vi "initialise variables.vi"(11 "Data in":T1={"Parameters"={"FPGA Ref"=refnum, "data stream"={"data writer name"="error writer", "NS write buffer size"=16, "NS Buffer length"=0}, "FIFO Depth"=0, "Channel controls"={"FIFO channel count"=0, "active indices"=[], "active channels"=0, "channelScaling"=[], "scanivalveCount"=0, "channels"=[]}, "safetyChannels"={"oilP"=0, "airP"=0, "water"=0, "channelLimits"=[]}, "speedChannel"=0, "maxSpeedLimit"=0.0, "Torque"={"fixedOffset"=0.0, "filter"=FALSE, "fallingEdge"=FALSE, "swapEncoders"=FALSE}}, "Variables"={"Intermediary buffer"=[], "buffer position"=0, "write loop counter"=0, "NS write trigger"=0, "NS Connection status"=FALSE, "waiting for NS"=FALSE, "labAmbient"={"pressure"=0.0, "temperature"=0.0}, "scanivalvePorts"=[], "scanivalvePressures"=[], "data stream"="", "activeChannelLimitIndex"=[], "runningSpeedLimit"=0.0, "speedChannelIndex"=0, "Interlocks"={"gearboxOil"=FALSE, "bearingOil"=FALSE, "gearboxAir"=FALSE}, "interlockChannels"={"gearboxOil"=0, "bearingOil"=0, "air"=0}, "limitStates"=[]}}) -> (3 "Data out":T1={"Parameters"={"FPGA Ref"=refnum, "data stream"={"data writer name"="error writer", "NS write buffer size"=16, "NS Buffer length"=0}, "FIFO Depth"=0, "Channel controls"={"FIFO channel count"=0, "active indices"=[], "active channels"=0, "channelScaling"=[], "scanivalveCount"=0, "channels"=[]}, "safetyChannels"={"oilP"=0, "airP"=0, "water"=0, "channelLimits"=[]}, "speedChannel"=0, "maxSpeedLimit"=0.0, "Torque"={"fixedOffset"=0.0, "filter"=FALSE, "fallingEdge"=FALSE, "swapEncoders"=FALSE}}, "Variables"={"Intermediary buffer"=[], "buffer position"=0, "write loop counter"=0, "NS write trigger"=0, "NS Connection status"=FALSE, "waiting for NS"=FALSE, "labAmbient"={"pressure"=0.0, "temperature"=0.0}, "scanivalvePorts"=[], "scanivalvePressures"=[], "data stream"="", "activeChannelLimitIndex"=[], "runningSpeedLimit"=0.0, "speedChannelIndex"=0, "Interlocks"={"gearboxOil"=FALSE, "bearingOil"=FALSE, "gearboxAir"=FALSE}, "interlockChannels"={"gearboxOil"=0, "bearingOil"=0, "air"=0}, "limitStates"=[]}})   [LabVIEW 2018]
uses:
  Type Defs/Data processing loop data.ctl
  Type Defs/FPGA reference.ctl
  PC/type defs/channelControl.ctl
  Type Defs/channelScalingTypes.ctl
  Type Defs/scalingMethods.ctl
  ICL-LabVIEW_General/data channels/parent class/Data Channel.lvclass
  PC/type defs/channelLimitControl.ctl
  PC/type defs/limitActions.ctl
  Type Defs/channelConfigFilePath.ctl
  ICL-LabVIEW_General/data channels/data channels.lvlib
types:
  T1 = typedef "Data processing loop data.ctl" = cluster{"Parameters":cluster{"FPGA Ref":T2, "data stream":cluster{"data writer name":string, "NS write buffer size":i32, "NS Buffer length":u32}, "FIFO Depth":u32, "Channel controls":cluster{"FIFO channel count":i32, "active indices":i16[], "active channels":i32, "channelScaling":T3[], "scanivalveCount":i32, "channels":refnum<class "Data Channel.lvclass">[]}, "safetyChannels":cluster{"oilP":u16, "airP":u16, "water":u16, "channelLimits":T6[]}, "speedChannel":i32, "maxSpeedLimit":dbl, "Torque":cluster{"fixedOffset":dbl, "filter":bool, "fallingEdge":bool, "swapEncoders":bool}}, "Variables":cluster{"Intermediary buffer":dbl[][], "buffer position":u32, "write loop counter":u16, "NS write trigger":u32, "NS Connection status":bool, "waiting for NS":bool, "labAmbient":cluster{"pressure":dbl, "temperature":dbl}, "scanivalvePorts":u16[], "scanivalvePressures":dbl[], "data stream":refnum<k21>, "activeChannelLimitIndex":u16[], "runningSpeedLimit":dbl, "speedChannelIndex":i32, "Interlocks":cluster{"gearboxOil":bool, "bearingOil":bool, "gearboxAir":bool}, "interlockChannels":cluster{"gearboxOil":i32, "bearingOil":i32, "air":i32}, "limitStates":cluster{"warn":bool, "alarm":bool}[]}}
  T2 = typedef "FPGA reference.ctl" = refnum<k20>
  T3 = typedef "channelControl.ctl" = cluster{"index":u16, "active":bool, "channelType":T4, "module":u16, "terminal":u16, "channelName":string, "scalingMethod":T5, "scalingParameters":dbl[], "scaledUnits":string, "tempOffset":dbl}
  T4 = typedef "channelScalingTypes.ctl" = enum16{"calculation", "measurement", "scanivalve", "output", "digital"}
  T5 = typedef "scalingMethods.ctl" = enum16{"none", "linear", "thermocouple", "polynomial", "encoder", "RTD"}
  T6 = typedef "channelLimitControl.ctl" = cluster{"channelID":u16, "Enabled":bool, "warnValue":dbl, "limitValue":dbl, "Invert":bool, "limitAction":T7}
  T7 = typedef "limitActions.ctl" = enum16{"stop", "shutdown", "ignore"}
  T8 = typedef "channelConfigFilePath.ctl" = path
  T9 = typedef "data channels.lvlib/Data Channel.lvclass/basic channel details.ctl" = cluster{"index":u16, "Active":bool, "channel name":string, "units":string, "module":string, "port":string, "liveOffset":dbl, "precision":u8, "channelType":T10, "fifoIndex":u16, "dataSource":T11, "acquireIndex":u16}
  T10 = typedef "data channels.lvlib/Data Channel.lvclass/channel type.ctl" = enum16{"acquisition", "output", "other"}
  T11 = typedef "data channels.lvlib/Data Channel.lvclass/dataSource.ctl" = enum16{"Not available", "FIFO", "Scanivalve", "Remote", "Calculated"}
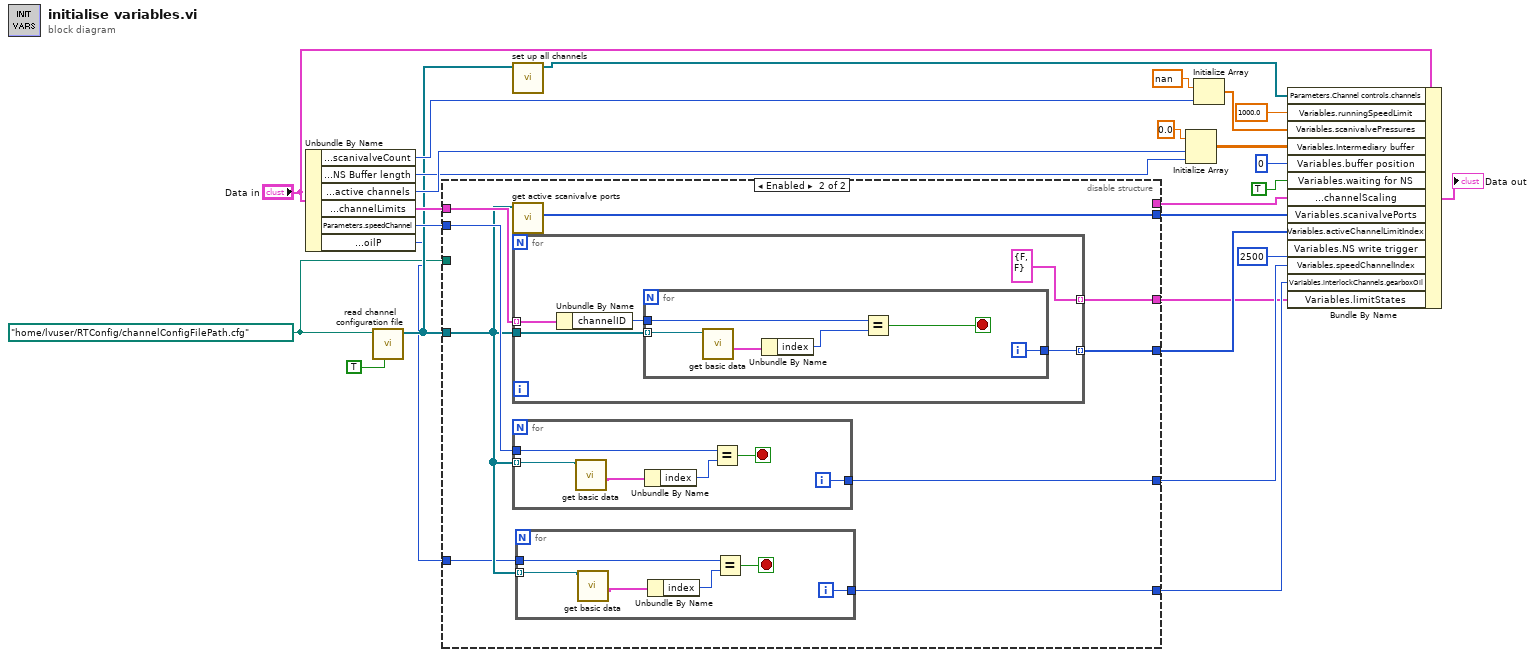
[diagram p0: block diagram]
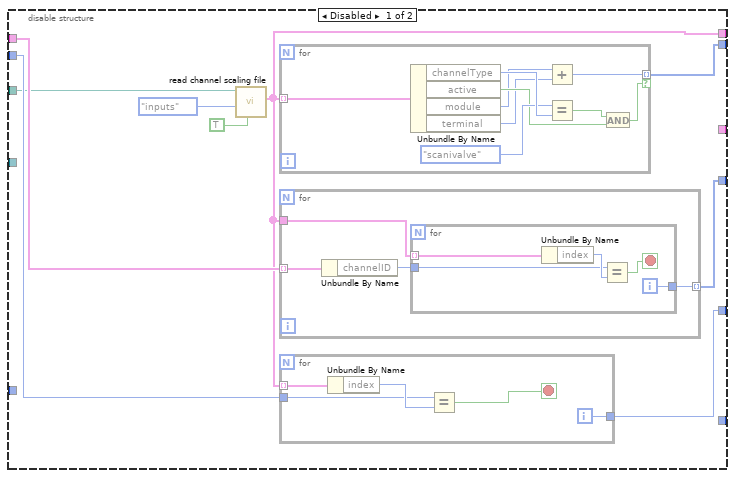
[diagram p2: hidden frame]
diagram:
  w5 = T8 path "/home/lvuser/RTConfig/channelConfigFilePath.cfg" ("channelConfigFilePath")
  n1 = Unbundle By Name("Data in") -> ("Parameters.Channel controls.scanivalveCount"=w15:i32, "Parameters.data stream.NS Buffer length"=w22:u32, "Parameters.Channel controls.active channels"=w23:i32, "Parameters.safetyChannels.channelLimits"=w14:T6[], "Parameters.speedChannel"=w10:i32, "Parameters.safetyChannels.oilP"=w3:u16)
  n2 = call "read channel configuration file.vi"("Hide inactive (F)"=TRUE, "config file"=w5) -> ("channelsArray"=w7:refnum<class "Data Channel.lvclass">[])  [unwired: 7 in, 2 out]
  n3 = disable-structure shown="Enabled" {
    disable-tunnel: [w35 w67] -> w18
    disable-tunnel: w14 -> [w34 w66]
    disable-tunnel: [w33 w65] -> w13
    disable-tunnel: w10 -> [w32 w64]
    disable-tunnel: [w31 w63] -> w9
    disable-tunnel: w7 -> [_ w62]
    disable-tunnel: w5 -> [w28 _]
    disable-tunnel: [w27 _] -> w4
    disable-tunnel: w3 -> [_ w61]
    disable-tunnel: [_ w60] -> w2
    disable-tunnel: [_ w59] -> w1
    frame Disabled {
      n4 = call "read channel scaling file.vi"("suppress inactive? (F)"=TRUE, "mode (all)"=enum16{"all", "inputs", "outputs", "digital"}."inputs", "file path"=w28) -> ("channelConfig"=w27:T3[])  [unwired: 4 in, 4 out]
      n5 = for {
        tunnel: w27 -> [w58] mode=indexing
        tunnel: [w53] -> w35 mode=indexing if=w52
        n6 = Unbundle By Name(w58) -> ("channelType"=w57:T4, "active"=w54:bool, "module"=w51:u16, "terminal"=w50:u16)
        n7 = Add(x=w51, y=w50) -> (x+y=w53:u16)
        n8 = Equal?(x=channelScalingTypes."scanivalve", y=w57) -> (x = y?=w55:bool)
        n9 = And(x=w55, y=w54) -> (x .and. y?=w52:bool)
      }
      n10 = for {
        tunnel: w34 -> [w44] mode=indexing
        tunnel: w27 -> [w42]
        tunnel: [w41] -> w33 mode=indexing
        n11 = Unbundle By Name(w44) -> ("channelID"=w43:u16)
        n12 = for {
          tunnel: w43 -> [w47]
          tunnel: w42 -> [w49] mode=indexing
          tunnel: [w46] -> w41
          i -> [w46]
          stop <- w45 stop-if-true
          n13 = Unbundle By Name(w49) -> ("index"=w48:u16)
          n14 = Equal?(x=w47, y=w48) -> (x = y?=w45:bool)
        }
      }
      n15 = for {
        tunnel: w32 -> [w38]
        tunnel: w27 -> [w40] mode=indexing
        tunnel: [w37] -> w31
        i -> [w37]
        stop <- w36 stop-if-true
        n16 = Unbundle By Name(w40) -> ("index"=w39:u16)
        n17 = Equal?(x=w38, y=w39) -> (x = y?=w36:bool)
      }
    }
    frame Enabled {
      n18 = call "get active scanivalve ports.vi"("channels"=w62) -> ("activeScanivalvePorts"=w67:i32[])  [unwired: 10 in]
      n19 = for {
        tunnel: w66 -> [w84] mode=indexing
        tunnel: [w82] -> w65 mode=indexing
        tunnel: w62 -> [w81]
        tunnel: [cluster{"warn":bool, "alarm":bool} {"warn"=FALSE, "alarm"=FALSE} ("limitStates")] -> w59 mode=indexing
        n20 = Unbundle By Name(w84) -> ("channelID"=w83:u16)
        n21 = for {
          tunnel: w83 -> [w90]
          tunnel: [w89] -> w82
          tunnel: w81 -> [w86] mode=indexing
          i -> [w89]
          stop <- w88 stop-if-true
          n22 = call "get basic data.vi"("Data Channel in"=w86) -> ("details"=w85:T9)  [unwired: 9 in, 1 out]
          n23 = Unbundle By Name(w85) -> ("index"=w87:u16)
          n24 = Equal?(x=w90, y=w87) -> (x = y?=w88:bool)
        }
      }
      n25 = for {
        tunnel: w64 -> [w79]
        tunnel: [w78] -> w63
        tunnel: w62 -> [w75] mode=indexing
        i -> [w78]
        stop <- w77 stop-if-true
        n26 = call "get basic data.vi"("Data Channel in"=w75) -> ("details"=w74:T9)  [unwired: 9 in, 1 out]
        n27 = Unbundle By Name(w74) -> ("index"=w76:u16)
        n28 = Equal?(x=w79, y=w76) -> (x = y?=w77:bool)
      }
      n29 = for {
        tunnel: w61 -> [w73]
        tunnel: [w72] -> w60
        tunnel: w62 -> [w69] mode=indexing
        i -> [w72]
        stop <- w71 stop-if-true
        n30 = call "get basic data.vi"("Data Channel in"=w69) -> ("details"=w68:T9)  [unwired: 9 in, 1 out]
        n31 = Unbundle By Name(w68) -> ("index"=w70:u16)
        n32 = Equal?(x=w73, y=w70) -> (x = y?=w71:bool)
      }
    }
  }
  n33 = call "set up all channels.vi"("channels"=w7) -> ("setUp channels"=w6:refnum<class "Data Channel.lvclass">[])  [unwired: 10 in]
  n34 = Initialize Array(sgl 0.0 ("element"), w23, w22) -> (w21:sgl[][])
  n35 = Initialize Array(sgl nan ("element"), w15) -> (w16:sgl[])
  n36 = Bundle By Name(cluster="Data in", "Parameters.Channel controls.channels"=w6, "Variables.runningSpeedLimit"=1000.0, "Variables.scanivalvePressures"=w16, "Variables.Intermediary buffer"=w21, "Variables.buffer position"=u32 0, "Variables.waiting for NS"=TRUE, "Parameters.Channel controls.channelScaling"=w4, "Variables.scanivalvePorts"=w18, "Variables.activeChannelLimitIndex"=w13, "Variables.NS write trigger"=u32 2500, "Variables.speedChannelIndex"=w9, "Variables.interlockChannels.gearboxOil"=w2, "Variables.limitStates"=w1) -> (→"Data out":T1)
